vi "TInitializePIStageOutput.vi"(1 "Image Settings":T1={"Start Position (µm)"={"x"=0.0, "y"=0.0, "z"=0.0}, "End Position (µm)"={"x"=10.0, "y"=10.0, "z"=0.0}, "Image Resolution (nm/pixel)"={"x"=50.0, "y"=50.0, "z"=100.0}, "Image Size (µm)"={"x"=10.0, "y"=10.0, "z"=0.0}, "Image Size (pixel)"={"x"=50, "y"=50, "z"=0}, "Time Resolution\n(ms/pixel)"=7.0, "1st Axis"=0, "2nd Axis"=1, "Retrace"=FALSE, "Estimated Time"=""} {"2nd Axis" items=["x", "y", "z"]; "1st Axis" items=["x", "y", "z"]; "Time Resolution\n(ms/pixel)" format="%.2f"; "Image Resolution (nm/pixel)"."z" format="%.2f"; "Image Resolution (nm/pixel)"."y" format="%.2f"; "Image Resolution (nm/pixel)"."x" format="%.2f"; "Image Size (µm)"."z" format="%.2f"; "Image Size (µm)"."y" format="%.2f"; "Image Size (µm)"."x" format="%.2f"; "End Position (µm)"."z" format="%.2f"; "End Position (µm)"."y" format="%.2f"; "End Position (µm)"."x" format="%.2f"; "Start Position (µm)"."z" format="%.2f"; "Start Position (µm)"."y" format="%.2f"; "Start Position (µm)"."x" format="%.2f"}, 2 "Timing Info":T2 {"#s" format="%.2f"; "Fs" format="%.2f"}) -> (0 "Analog Output":T3)   [LabVIEW 2009]
uses:
  AnalogTrace.ctt
  TimingInfo.ctt
  ImageSettings.ctt
panel:
  out "Waveform Graph":dbl[](graph)
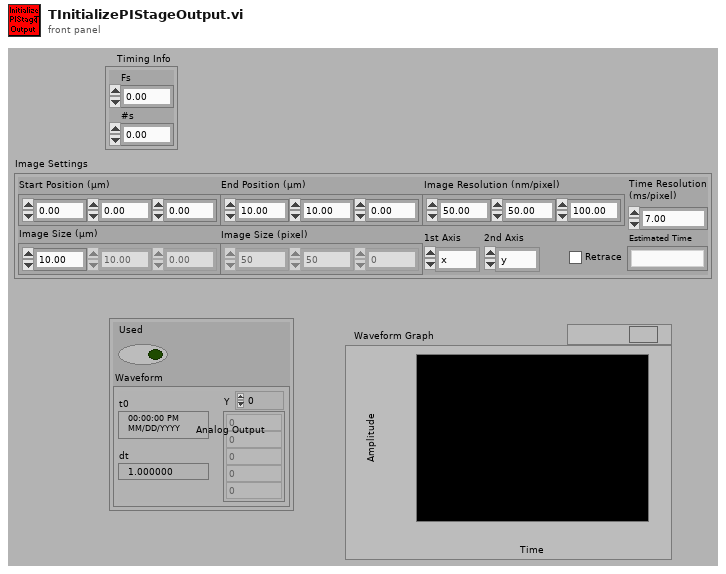
[diagram p1: front panel]
types:
  T1 = typedef "ImageSettings.ctt" = cluster{"Start Position (µm)":cluster{"x":dbl, "y":dbl, "z":dbl}, "End Position (µm)":cluster{"x":dbl, "y":dbl, "z":dbl}, "Image Resolution (nm/pixel)":cluster{"x":dbl, "y":dbl, "z":dbl}, "Image Size (µm)":cluster{"x":dbl, "y":dbl, "z":dbl}, "Image Size (pixel)":cluster{"x":u32, "y":u32, "z":u32}, "Time Resolution\n(ms/pixel)":dbl, "1st Axis":u16, "2nd Axis":u16, "Retrace":bool, "Estimated Time":string}
  T2 = typedef "TimingInfo.ctt" = cluster{"Fs":dbl, "#s":dbl}
  T3 = typedef "AnalogTrace.ctt" = cluster{"Used":bool, "Waveform":waveform(dbl)}
  T4 = typedef "StageSettings.ctt" = cluster{"channels (x, y, z)":tag, "Stage Scaling (V/µm)":dbl}
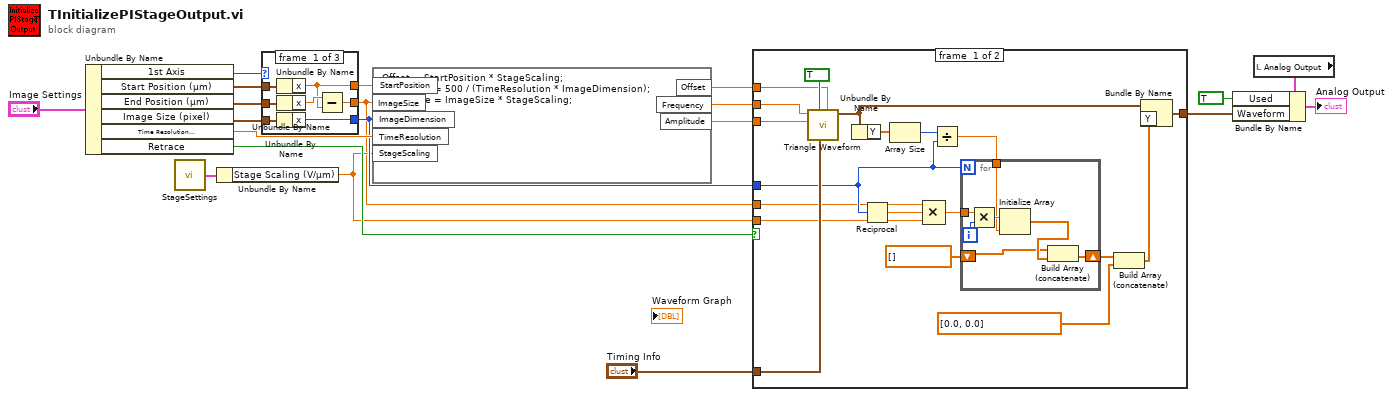
[diagram p0: block diagram]
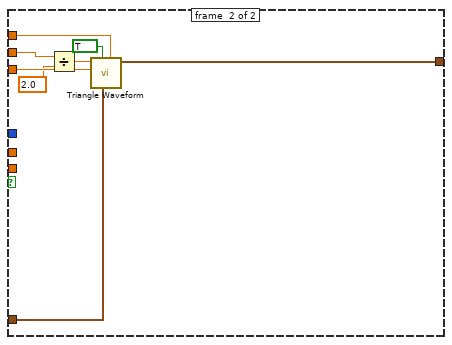
[diagram p2: hidden frame]
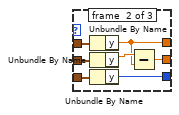
[diagram p3: hidden frame]
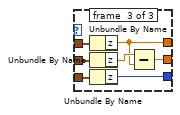
[diagram p4: hidden frame]
diagram:
  n1 = Unbundle By Name("Image Settings") -> ("1st Axis"=w11:u16, "Start Position (µm)"=w10:cluster{"x":dbl, "y":dbl, "z":dbl}, "End Position (µm)"=w8:cluster{"x":dbl, "y":dbl, "z":dbl}, "Image Size (pixel)"=w7:cluster{"x":u32, "y":u32, "z":u32}, "Time Resolution\n(ms/pixel)"=w9:dbl, "Retrace"=w6:bool)
  n2 = call "StageSettings.vi"() -> ("PI Stage Setup (output)"=w20:T4)  [unwired: 2 in]
  n3 = Unbundle By Name(w20) -> ("Stage Scaling (V/µm)"=w2:dbl)
  n4 = case shown="0, Default" w11 {
    tunnel: w10 -> [w27 w34 w41]
    tunnel: [w21 w28 w35] -> w19
    tunnel: w8 -> [w26 w33 w40]
    tunnel: [w23 w30 w37] -> w1
    tunnel: w7 -> [w25 w32 w39]
    tunnel: [w24 w31 w38] -> w3
    frame #0 {
      n5 = Unbundle By Name(w27) -> ("x"=w21:dbl)
      n6 = Unbundle By Name(w26) -> ("x"=w22:dbl)
      n7 = Unbundle By Name(w25) -> ("x"=w24:u32)
      n8 = Subtract(x=w22, y=w21) -> (x-y=w23:dbl)
    }
    frame #1 {
      n9 = Unbundle By Name(w34) -> ("y"=w28:dbl)
      n10 = Unbundle By Name(w33) -> ("y"=w29:dbl)
      n11 = Unbundle By Name(w32) -> ("y"=w31:u32)
      n12 = Subtract(x=w29, y=w28) -> (x-y=w30:dbl)
    }
    frame #2 {
      n13 = Unbundle By Name(w41) -> ("z"=w35:dbl)
      n14 = Unbundle By Name(w40) -> ("z"=w36:dbl)
      n15 = Unbundle By Name(w39) -> ("z"=w38:u32)
      n16 = Subtract(x=w36, y=w35) -> (x-y=w37:dbl)
    }
  }
  n17 = formula code="Offset = StartPosition * StageScaling;\nFrequency = 500 / (TimeResolution * ImageDimension);\nAmplitude = ImageSize * StageScaling;"("StartPosition"=w19, "ImageDimension"=w3, "ImageSize"=w1, "TimeResolution"=w9, "StageScaling"=w2) -> ("Offset"=w18:dbl, "Frequency"=w17:dbl, "Amplitude"=w16:dbl)
  n18 = case shown="False" w6 {
    tunnel: w18 -> [w59 w75]
    tunnel: w17 -> [w45 w69]
    tunnel: w16 -> [w58 w73]
    tunnel: [w49 w72] -> w5
    tunnel: "Timing Info" -> [w57 w71]
    tunnel: w3 -> [w48 _]
    tunnel: w2 -> [w47 _]
    tunnel: w1 -> [w46 _]
    frame #0 {
      n19 = call "Triangle Waveform.vi"("offset"=w59, "sampling info"=w57, "reset signal"=TRUE, "amplitude"=w58, "frequency"=w45) -> ("signal out"=w50:waveform(dbl))  [unwired: 5 in, 1 out]
      n20 = Unbundle By Name(w50) -> ("Y"=w52:dbl[])
      n21 = Reciprocal(x=w48) -> (1/x=w53:dbl)
      n22 = Array Size(array=w52) -> (size(s)=w51:i32)
      n23 = Compound Arithmetic op=MULTIPLY(w46, w53, w47) -> (w55:dbl)
      n24 = Divide(x=w51, y=w48) -> (x/y=w56:dbl)
      n25 = for {
        N: w48 -> [_]
        tunnel: w56 -> [w64]
        tunnel: w55 -> [w67]
        shift-right: [w61] -> w44
        shift-left: dbl[] [] -> [w62]
        i -> [w66]
        n26 = Multiply(x=w67, y=w66) -> (x*y=w65:dbl)
        n27 = Initialize Array(w65, w64) -> (w63:dbl[])
        n28 = Build Array (concatenate)(w62, w63) -> (w61:dbl[])
      }
      n29 = Build Array (concatenate)(w44, dbl[] [0.0, 0.0] ("array")) -> (w43:dbl[])
      n30 = Bundle By Name(cluster=w50, "Y"=w43) -> (w49:waveform(dbl))
    }
    frame #1 {
      n31 = Divide(x=w69, y=2.0) -> (x/y=w70:dbl)
      n32 = call "Triangle Waveform.vi"("offset"=w75, "sampling info"=w71, "reset signal"=TRUE, "amplitude"=w73, "frequency"=w70) -> ("signal out"=w72:waveform(dbl))  [unwired: 5 in, 1 out]
    }
  }
  n33 = local read "Analog Output"() -> (w13:T3)
  n34 = Bundle By Name(cluster=w13, "Used"=TRUE, "Waveform"=w5) -> (→"Analog Output":T3)
